vi "Cleanup.vi"(0 "Detected Type":T1, 1 "MetaDataObj in":refnum<class "MetaDataObj.lvclass">, 5 "UI Ref Cluster":T3, 7 "Target Info":T2[](array[typedef]) {"ProdID" format="%.0x"}, 9 "Supported Devices":u32[](array[numeric]), 11 "error in":errorcluster, 12 "Target FPGA Personality":string, 13 "Owning VI Ref":refnum<vi>) -> (3 "MetaDataObj out":refnum<class "MetaDataObj.lvclass">, 15 "error out":errorcluster)   [LabVIEW 2021, in "myRIOMetaDataObj.lvclass"]
uses:
  myRIOMetaDataObj.lvclass
  WizardUIRef.ctl
  AvailableTargets.ctl
  <resource>/myRIO/Target Info.ctl
  <resource>/dialog/NewProjectWizard/MetaDataObj/MetaDataObj.lvclass
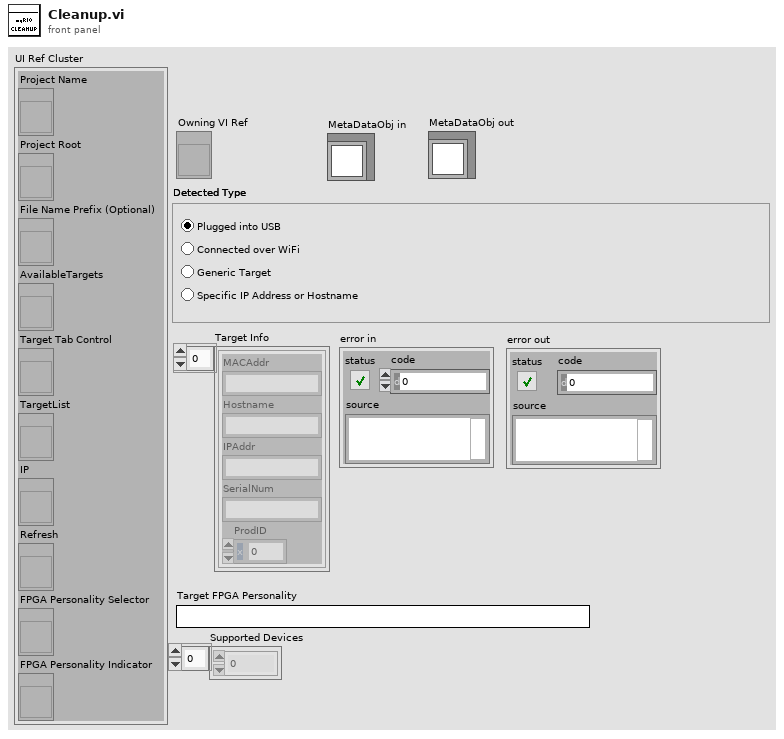
[diagram p1: front panel]
types:
  T1 = typedef "myRIOMetaDataObj.lvclass/AvailableTargets.ctl" = enum32{"USBTarget", "WifiTarget", "NoSpecificTarget", "TargetIP"}
  T2 = typedef "Target Info.ctl" = cluster{"MACAddr":string, "Hostname":string, "IPAddr":string, "SerialNum":string, "ProdID":u32}
  T3 = typedef "myRIOMetaDataObj.lvclass/WizardUIRef.ctl" = cluster{"Project Name":refnum<vi>, "Project Root":refnum<vi>, "File Name Prefix (Optional)":refnum<vi>, "AvailableTargets":refnum<vi>, "Target Tab Control":refnum<vi>, "TargetList":refnum<vi>, "IP":refnum<vi>, "Refresh":refnum<vi>, "FPGA Personality Selector":refnum<vi>, "FPGA Personality Indicator":refnum<vi>}
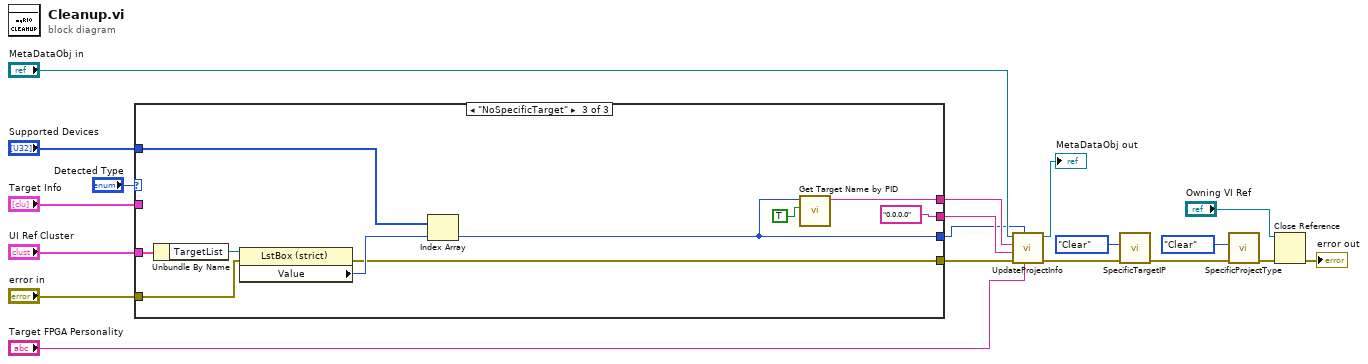
[diagram p0: block diagram]
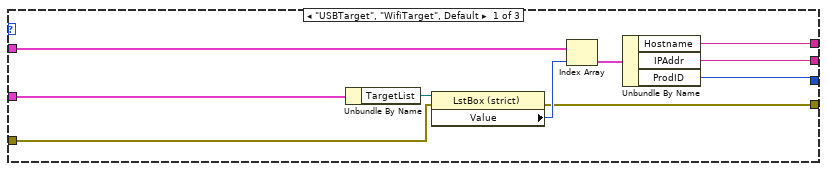
[diagram p2: hidden frame]
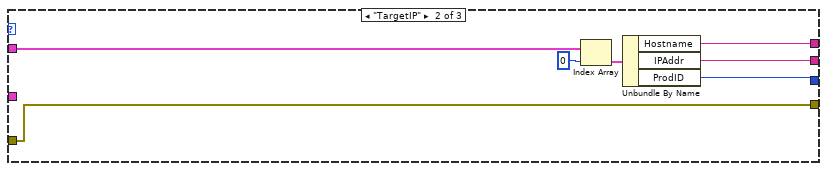
[diagram p3: hidden frame]
diagram:
  n1 = case shown="\"NoSpecificTarget\"" "Detected Type" {
    tunnel: [w27 w34 w38] -> w18
    tunnel: [w26 w33 "0.0.0.0"] -> w17
    tunnel: [w22 w30 w40] -> w19
    tunnel: [w21 w31 w39] -> w1
    tunnel: "UI Ref Cluster" -> [w25 _ w44]
    tunnel: "Target Info" -> [w23 w32 _]
    tunnel: "Supported Devices" -> [_ _ w42]
    tunnel: "error in" -> [w20 w30 w41]
    frame "USBTarget", "WifiTarget", Default {
      n2 = Unbundle By Name(w25) -> ("TargetList"=w24:refnum<vi>)
      n3 = property class="LstBox (strict)"(reference=w24, error in=w20) -> (error out=w22:errorcluster, "Value"=w29:i32)  [unwired: 1 out]
      n4 = Index Array(array=w23, index=w29) -> (element=w28:T2)
      n5 = Unbundle By Name(w28) -> ("Hostname"=w27:string, "IPAddr"=w26:string, "ProdID"=w21:u32)
    }
    frame "TargetIP" {
      n6 = Index Array(array=w32, index=0) -> (element=w35:T2)
      n7 = Unbundle By Name(w35) -> ("Hostname"=w34:string, "IPAddr"=w33:string, "ProdID"=w31:u32)
    }
    frame "NoSpecificTarget" {
      n8 = Unbundle By Name(w44) -> ("TargetList"=w43:refnum<vi>)
      n9 = property class="LstBox (strict)"(reference=w43, error in=w41) -> (error out=w40:errorcluster, "Value"=w45:i32)  [unwired: 1 out]
      n10 = Index Array(array=w42, index=w45) -> (element=w39:u32)
      n11 = call <vilib>:"Get Target Name by PID.vi"("Full Name?"=TRUE, "Device Model"=w39) -> ("Device Model Str"=w38:string)  [unwired: 8 in, 1 out]
    }
  }
  n12 = call "UpdateProjectInfo.vi"("Target FPGA Personality"="Target FPGA Personality", "Device Code"=w1, "error in (no error)"=w19, "Target Address"=w17, "Target Name"=w18, "MetaDataObj in"="MetaDataObj in") -> ("error out"=w16:errorcluster, "MetaDataObj out"=→"MetaDataObj out":refnum<class "MetaDataObj.lvclass">)  [unwired: 4 in]
  n13 = call "SpecificTargetIP.vi"("error in (no error)"=w16, "Action"=enum16{"Clear", "Get", "Set"}."Clear") -> ("error out"=w14:errorcluster)  [unwired: 8 in, 1 out]
  n14 = call "SpecificProjectType.vi"("error in (no error)"=w14, "Action"=enum16{"Clear", "Get", "Set"}."Clear") -> ("error out"=w12:errorcluster)  [unwired: 6 in, 3 out]
  n15 = Close Reference(reference="Owning VI Ref", error in (no error)=w12) -> (error out=→"error out":errorcluster)
